vi "SetContinuousMeasurement.vi"(8 "error in (no error)":errorcluster, 11 "on":bool) -> (0 "error out":errorcluster)   [LabVIEW 2015, in "ESLSCDLL.lvlib"]
uses:
  ESLSCDLL.lvlib
  Globals.vi
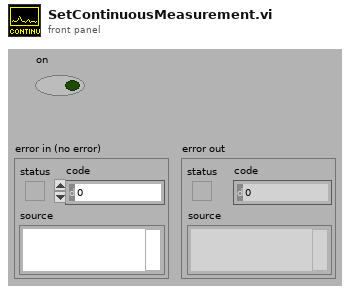
[diagram p1: front panel]
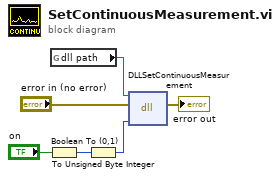
[diagram p0: block diagram]
diagram:
  n1 = Boolean To (0,1)(Boolean="on") -> (0, 1=w3:i16)
  n2 = global read "Globals.vi" "dll path"() -> (w1:path)
  n3 = To Unsigned Byte Integer(number=w3) -> (unsigned 8bit integer=w5:u8)
  n4 = dll-call lib="C:/ENTW/PCIE/LV64/board.vis/ESLSCDLL.dll" fn="DLLSetContinuousMeasurement" ("lwlscdll.dll:DLLRsTOREG")(path in=w1, error in="error in (no error)", "on"=w5) -> (error out=→"error out":errorcluster)  [unwired: 3 in, 1 out]
